vi "ENA_Display On_Off.vi"(0 "Semiconductor Module Context":T1, 5 "Pins":string[](array[string])=["RF1", "RF2"], 7 "ENA Display Mode":enum16{"ON", "OFF"}(ring), 11 "error in (no error)":errorcluster) -> (6 "Semiconductor Module Context Out":T1, 15 "error out":errorcluster)   [LabVIEW 2013]
uses:
  <vilib>/NI_TestStand_SemiconductorModule/NI_TestStand_Semiconductor_Module.lvlibp/PinMap/General/SemiconductorModuleContext.ctl
  Pin Map API/ENA Custom Instrument.lvlib
  <vilib>/NI_TestStand_SemiconductorModule/NI_TestStand_Semiconductor_Module.lvlibp
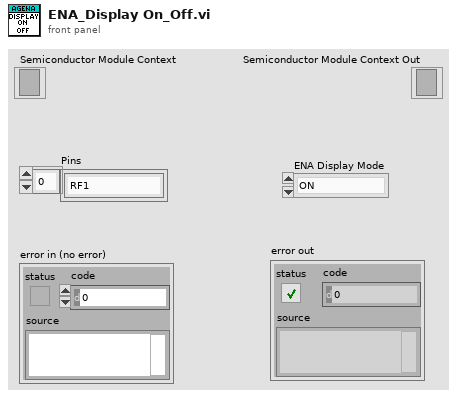
[diagram p1: front panel]
types:
  T1 = typedef "NI_TestStand_Semiconductor_Module.lvlibp/SemiconductorModuleContext.ctl" = refnum<k7>
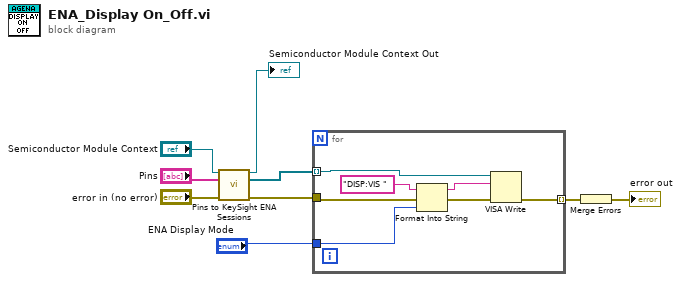
[diagram p0: block diagram]
diagram:
  n1 = call "Pins to KeySight ENA Sessions.vi"("Semiconductor Module Context"="Semiconductor Module Context", "Pins"="Pins", "error in (no error)"="error in (no error)") -> ("Semiconductor Module Context Out"=→"Semiconductor Module Context Out":T1, "Instrument Sessions"=w7:refnum<visa-resource-name>[], "error out"=w8:errorcluster)  [unwired: 8 in, 2 out]
  n2 = for {
    tunnel: w7 -> [w10] mode=indexing
    tunnel: w8 -> [w13]
    tunnel: "ENA Display Mode" -> [w12]
    tunnel: [w11] -> w2 mode=indexing
    n3 = Format Into String(initial string="DISP:VIS " ("write buffer"), error in=w13, w12) -> (resulting string=w16:string, error out=w15:errorcluster)  [unwired: 1 in]
    n4 = VISA Write(VISA resource name=w10, write buffer=w16, error in (no error)=w15) -> (error out=w11:errorcluster)  [unwired: 2 out]
  }
  n5 = Merge Errors(w2) -> (→"error out":errorcluster)
